vi "Configure Vacuum Test.vi"(8 "error in (no error)":errorcluster, 11 "Test":string="G") -> (0 "error out":errorcluster)   [LabVIEW 2015]
panel:
  in  "Thresholds":i32(listbox)=-1
  in  "Timing":i32(listbox)=-2
  out "Cancelled?":bool
  in  "Cancel Button":bool
  in  "OK Button":bool
  out "Test Sequence":i32(listbox)=-2
  # "Configure Vacuum Test"
  # "Duration refers to the run time of each step\n\nPump ON refers to the time period that the pump is ON in each step"
  # "Each step may have a functionality test and/or a leak test\n\nA functionality test is conducted by obtaining a pressure reading (PSI) and determining whether it lies between a threshold window (Func P Max and Func P Min). \n\nA leak test is conducted by obtaining the leak rate of the pressure (PSI/s) and determining whether it lies between a threshold window (Leak P Max and Leak P Min)."
  # "For a threshold that does\nnot apply, please enter N/A"
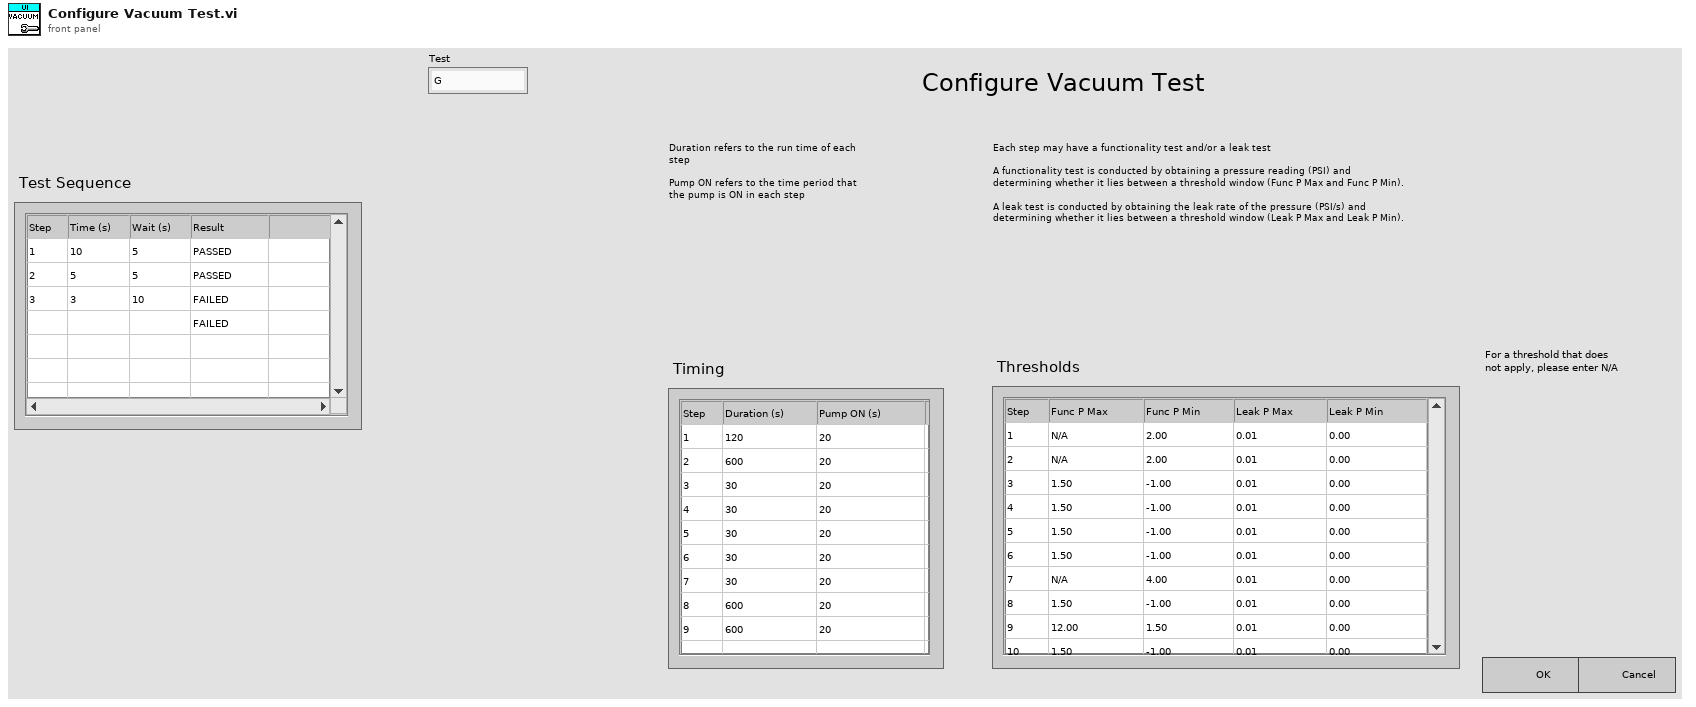
[diagram p1: front panel]
types:
  T1 = typedef "Test Configuration.ctl" = cluster{"GC":T2, "GC+EX":T2, "GC+EX+CMS":T2}
  T2 = typedef "Test Information.ctl" = cluster{"Vacuum Test":T3, "Helium Test":T6}
  T3 = typedef "Vacuum Test.ctl" = cluster{"Vacuum Timings":T4[], "Vacuum Thresholds":T5[], "Leak Reasons":string[], "Func Reasons":string[], "FuncSpecEqual":string[], "LeakSpecEqual":string[]}
  T4 = typedef "Test Timing.ctl" = cluster{"Step Wait":dbl, "Pump Wait":dbl}
  T5 = typedef "Vaccum Thresholds.ctl" = cluster{"Func Max Pressure":dbl, "Func Min Pressure":dbl, "Leak Max Pressure":dbl, "Leak Min Pressure":dbl}
  T6 = typedef "Helium Test.ctl" = cluster{"Helium Timings":T4[], "Helium Thresholds":T7[], "Failure Reasons":string[], "LeakSpecEqual":string[]}
  T7 = typedef "Helium Thresholds.ctl" = cluster{"Leak Max Pressure":dbl, "Leak Min Pressure":dbl}
  T8 = typedef "LVPoint32TypeDef.ctl" = cluster{"Horizontal":i32, "Vertical":i32}
  T9 = typedef "LVRowAndColumnTypeDef.ctl" = cluster{"Row":i32, "Column":i32}
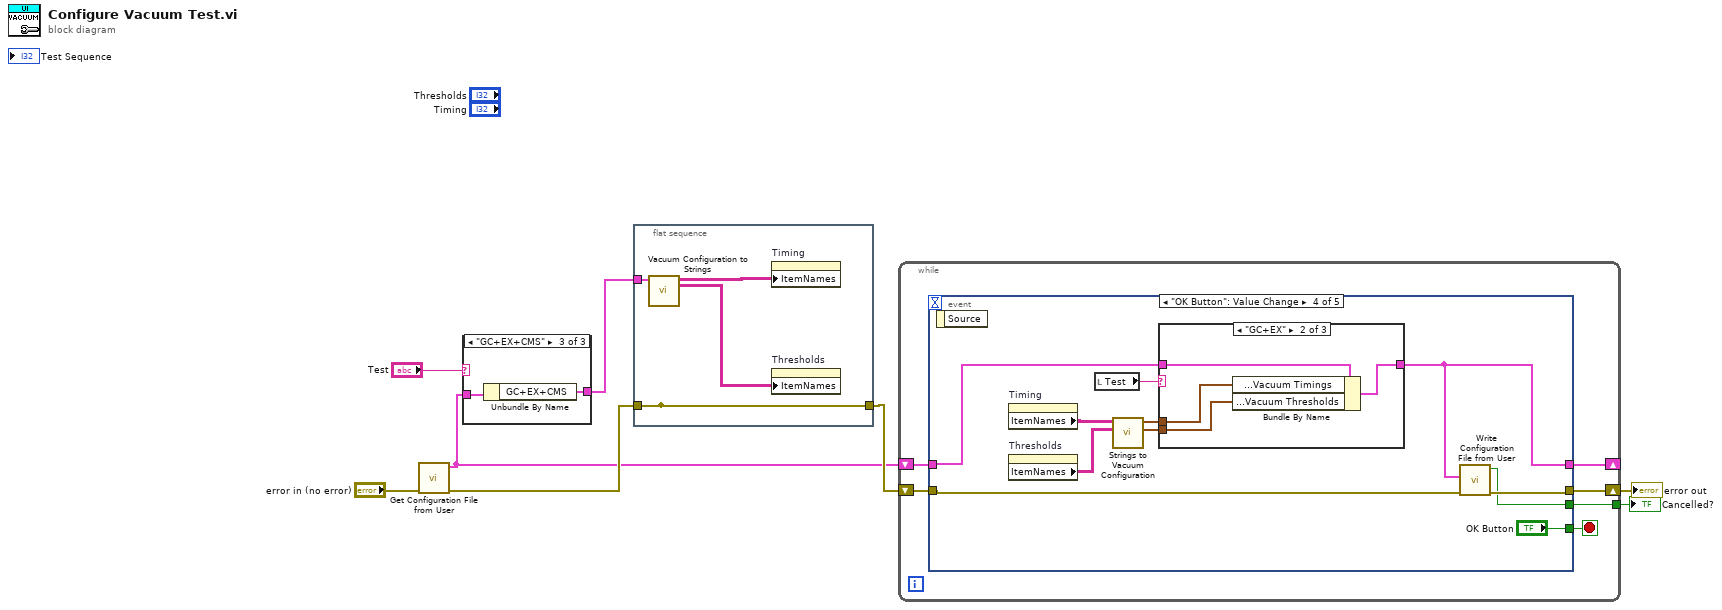
[diagram p0: block diagram]
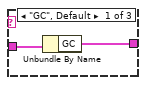
[diagram p2: hidden frame]
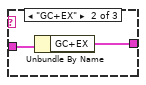
[diagram p3: hidden frame]
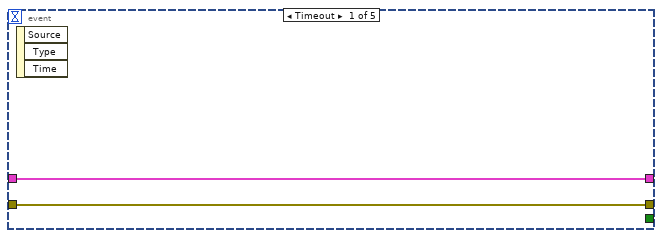
[diagram p4: hidden frame]
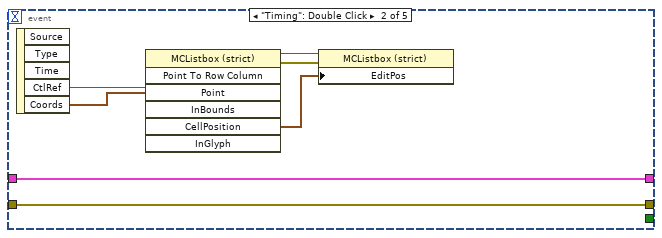
[diagram p5: hidden frame]
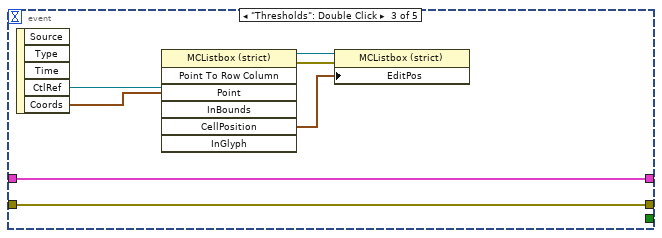
[diagram p6: hidden frame]
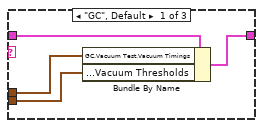
[diagram p7: hidden frame]
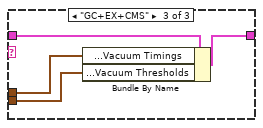
[diagram p8: hidden frame]
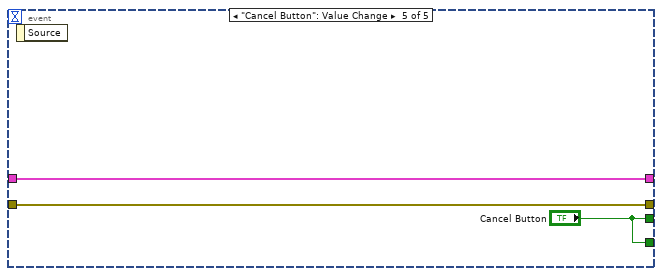
[diagram p9: hidden frame]
diagram:
  n1 = call "Get Configuration File from User.vi"("error in"="error in (no error)") -> ("error out"=w4:errorcluster, "Test Configuration"=w1:T1)  [unwired: 8 in, 1 out]
  n2 = case shown="\"GC+EX+CMS\"" "Test" {
    tunnel: w1 -> [w10 w12 w14]
    tunnel: [w9 w11 w13] -> w2
    frame "GC", Default {
      n3 = Unbundle By Name(w10) -> ("GC"=w9:T2)
    }
    frame "GC+EX" {
      n4 = Unbundle By Name(w12) -> ("GC+EX"=w11:T2)
    }
    frame "GC+EX+CMS" {
      n5 = Unbundle By Name(w14) -> ("GC+EX+CMS"=w13:T2)
    }
  }
  n6 = flat-sequence {
    tunnel: w2 -> [w16]
    tunnel: w4 -> [w15]
    tunnel: [w15] -> _
    tunnel: [w15] -> w3
    frame #0 {
      n7 = call "Vacuum Configuration to Strings.vi"("Test Information"=w16) -> ("Thresholds"=w17:string[][], "Timings"=w18:string[][])  [unwired: 9 in]
      n8 = property on="Timing" class="MCListbox (strict)"("ItemNames"=w18) -> ()  [unwired: 2 in, 2 out]
      n9 = property on="Thresholds" class="MCListbox (strict)"("ItemNames"=w17) -> ()  [unwired: 2 in, 2 out]
    }
  }
  n10 = while {
    tunnel: [w24] -> w8
    shift-right: [w21] -> w7
    shift-left: w3 -> [w22]
    shift-right: [w19] -> _
    shift-left: w1 -> [w20]
    stop <- w23 stop-if-true
    n11 = event shown="[3] \"OK Button\": Value Change" {
      selector: _ -> [_ _ _ _ _]
      dyn-events: _ -> [_ _ _ _ _]
      timeout: _ -> [_ _ _ _ _]
      tunnel: [_ _ _ w41 "Cancel Button"] -> w24
      tunnel: [_ _ _ "OK Button" "Cancel Button"] -> w23
      tunnel: w22 -> [w26 w28 w35 w47 w65]
      tunnel: [w26 w28 w35 w50 w65] -> w21
      tunnel: w20 -> [w25 w27 w34 w46 w64]
      tunnel: [w25 w27 w34 w42 w64] -> w19
      event Timeout {
        n12 = event-data() -> ()  [unwired: 1 in, 3 out]
      }
      event "Timing": Double Click {
        n13 = event-data() -> ("CtlRef"=w33:refnum<vi>, "Coords"=w32:T8)  [unwired: 1 in, 3 out]
        n14 = invoke class="MCListbox (strict)" method="Point To Row Column"(reference=w33, "Point"=w32) -> (reference out=w31:refnum<vi>, error out=w30:errorcluster, "CellPosition"=w29:T9)  [unwired: 5 in, 4 out]
        n15 = property class="MCListbox (strict)"(reference=w31, error in=w30, "EditPos"=w29) -> ()  [unwired: 2 out]
      }
      event "Thresholds": Double Click {
        n16 = event-data() -> ("CtlRef"=w40:refnum<vi>, "Coords"=w39:T8)  [unwired: 1 in, 3 out]
        n17 = invoke class="MCListbox (strict)" method="Point To Row Column"(reference=w40, "Point"=w39) -> (reference out=w38:refnum<vi>, error out=w37:errorcluster, "CellPosition"=w36:T9)  [unwired: 5 in, 4 out]
        n18 = property class="MCListbox (strict)"(reference=w38, error in=w37, "EditPos"=w36) -> ()  [unwired: 2 out]
      }
      event "OK Button": Value Change {
        n19 = event-data() -> ()  [unwired: 1 in, 1 out]
        n20 = property on="Timing" class="MCListbox (strict)"() -> ("ItemNames"=w49:string[][])  [unwired: 2 in, 2 out]
        n21 = property on="Thresholds" class="MCListbox (strict)"() -> ("ItemNames"=w48:string[][])  [unwired: 2 in, 2 out]
        n22 = local read "Test"() -> (w45:string)
        n23 = call "Strings to Vacuum Configuration.vi"("Thresholds"=w48, "Timings"=w49) -> ("Thresholds"=w43:T5[], "Timings"=w44:T4[])  [unwired: 8 in]
        n24 = case shown="\"GC+EX\"" w45 {
          tunnel: w46 -> [w55 w59 w63]
          tunnel: w44 -> [w54 w58 w62]
          tunnel: w43 -> [w53 w57 w61]
          tunnel: [w52 w56 w60] -> w42
          frame "GC", Default {
            n25 = Bundle By Name(cluster=w55, "GC.Vacuum Test.Vacuum Timings"=w54, "GC.Vacuum Test.Vacuum Thresholds"=w53) -> (w52:T1)
          }
          frame "GC+EX" {
            n26 = Bundle By Name(cluster=w59, "GC+EX.Vacuum Test.Vacuum Timings"=w58, "GC+EX.Vacuum Test.Vacuum Thresholds"=w57) -> (w56:T1)
          }
          frame "GC+EX+CMS" {
            n27 = Bundle By Name(cluster=w63, "GC+EX+CMS.Vacuum Test.Vacuum Timings"=w62, "GC+EX+CMS.Vacuum Test.Vacuum Thresholds"=w61) -> (w60:T1)
          }
        }
        n28 = call "Write Configuration File from User.vi"("error in"=w47, "Test Configuration"=w42) -> ("error out"=w50:errorcluster, "Cancelled?"=w41:bool)  [unwired: 8 in]
      }
      event "Cancel Button": Value Change {
        n29 = event-data() -> ()  [unwired: 1 in, 1 out]
      }
    }
  }
  "error out" <- w7
  "Cancelled?" <- w8
